vi "Delete Zero Rows in Array.vi"(9 "Array Size":i32, 10 "Initialized Array":sgl[][](array[numeric]), 11 "Sorted 2D array":sgl[][](array[numeric])) -> (0 "Boolean":bool, 3 "Array out":sgl[][](array[numeric]))   [LabVIEW 2020]
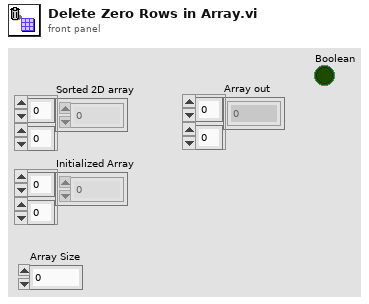
[diagram p1: front panel]
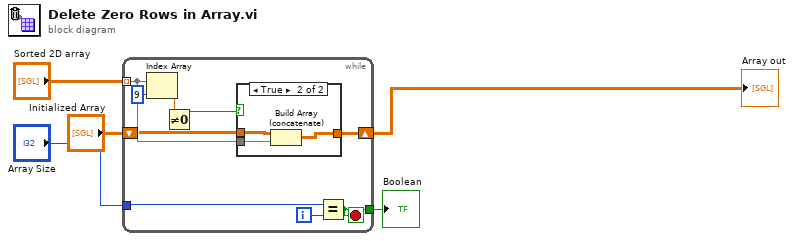
[diagram p0: block diagram]
diagram:
  n1 = while {
    tunnel: "Sorted 2D array" -> [w11] mode=indexing
    shift-right: [w10] -> w5
    shift-left: "Initialized Array" -> [w9]
    tunnel: "Array Size" -> [w7]
    tunnel: [w6] -> w1
    i -> [w8]
    stop <- w6 stop-if-true
    n2 = Index Array(array=w11, index=9) -> (element=w13:sgl)
    n3 = Not Equal To 0?(x=w13) -> (x != 0?=w12:bool)
    n4 = case shown="True" w12 {
      tunnel: w11 -> [_ w18]
      tunnel: [w15 w17] -> w10
      tunnel: w9 -> [w15 w16]
      frame False {
      }
      frame True {
        n5 = Build Array (concatenate)(w16, w18) -> (w17:sgl[][])
      }
    }
    n6 = Equal?(x=w7, y=w8) -> (x = y?=w6:bool)
  }
  "Array out" <- w5
  "Boolean" <- w1
